vi "FPGA Main Default.vi"() -> ()   [LabVIEW 2019]
doc: "The myRIO v1.1 FPGA Shipping Personality. This personality contains support for:\n- 2 Analog Input Interrupt channel\n- 4 Digital Input Interrupt channel\n- 1 Timer\n- 1 Accelerometer\n- 1 Button\n- 4 LED\n- 10 Analog Input channels with 1 Sample\n- 6 Analog Output channels with 1 Sample\n- 40 Digital I/O channels with 1 Sample\n- 2 I2C channels\n- 4 Encoder channels\n- 6 PWM channels\n- 2 SPI channels"
uses:
  <vilib>/rvi/Emulation/niFpgaGetClockAttributes.vi
  <vilib>/rvi/Emulation/niFpgaSctlEmulationGetInTimedLoop.vi
  <vilib>/rvi/Emulation/niFpgaEmulationReportErrorSimple.vi
  <vilib>/rvi/Emulation/niFpgaProcessEmulError.vi
  <vilib>/rvi/eio/common/nirviEmuTemplateMethod_errors.vi
  <vilib>/rvi/Emulation/niFpgaCriticalErrorInLSC.vi
  <vilib>/eio/EIONode/EIONode.xnode
panel:
  in  "BreakinLoop":bool
  in  "OFFTime":u32
  in  "ONTime":u32
  in  "Trigger":u64
  in  "PulseNumberperLoop":i32
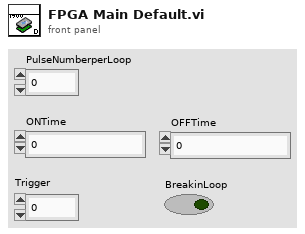
[diagram p1: front panel]
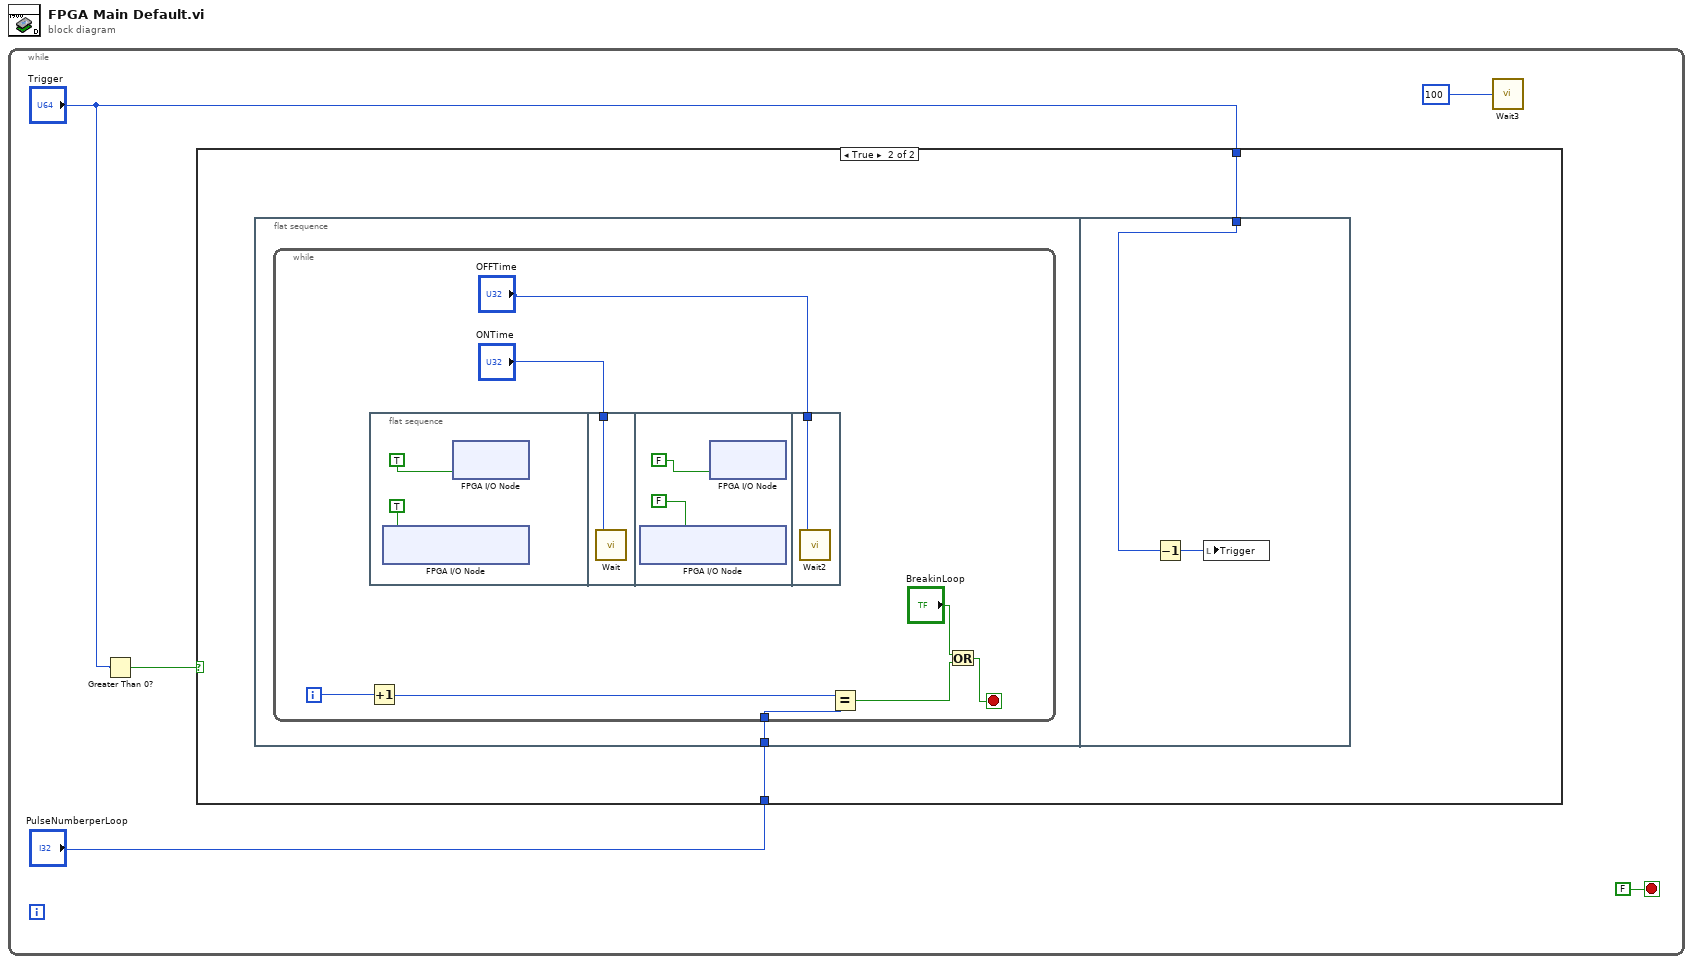
[diagram p0: block diagram]
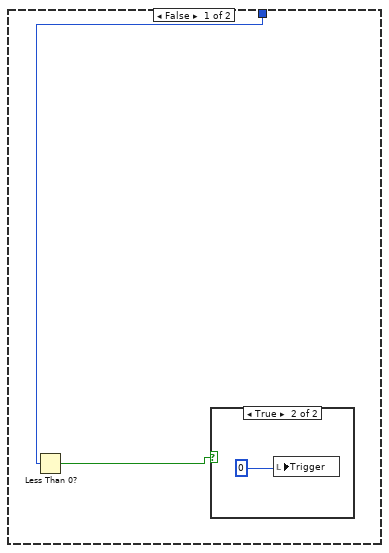
[diagram p2: hidden frame]
diagram:
  n1 = while {
    stop <- FALSE stop-if-true
    n2 = Greater Than 0?(x="Trigger") -> (x > 0?=w3:bool)
    n3 = case shown="True" w3 {
      tunnel: "PulseNumberperLoop" -> [_ w10]
      tunnel: "Trigger" -> [w7 w9]
      frame False {
        n4 = Less Than 0?(x=w7) -> (x < 0?=w6:bool)
        n5 = case shown="True" w6 {
          frame False {
          }
          frame True {
            n6 = local write "Trigger"(i16 0) -> ()
          }
        }
      }
      frame True {
        n7 = flat-sequence {
          tunnel: w10 -> [w11]
          tunnel: w9 -> [w26]
          frame #0 {
            n8 = while {
              tunnel: w11 -> [w12]
              i -> [w13]
              stop <- w17 stop-if-true
              n9 = Increment(x=w13) -> (x+1=w14:i32)
              n10 = flat-sequence {
                tunnel: "ONTime" -> [w22]
                tunnel: "OFFTime" -> [w25]
                frame #0 {
                  n11 = xnode "FPGA I/O Node"("ConnectorA/DIO8"=TRUE) -> ()  [unwired: 1 in, 1 out]
                  n12 = xnode "FPGA I/O Node"("LED0"=TRUE ("ConnectorA/DIO8")) -> ()  [unwired: 1 in, 1 out]
                }
                frame #1 {
                  n13 = call "Wait"("Count(uSec)"=w22) -> ()  [unwired: 1 out]
                }
                frame #2 {
                  n14 = xnode "FPGA I/O Node"("ConnectorA/DIO8"=FALSE) -> ()  [unwired: 1 in, 1 out]
                  n15 = xnode "FPGA I/O Node"("LED0"=FALSE ("ConnectorA/DIO8")) -> ()  [unwired: 1 in, 1 out]
                }
                frame #3 {
                  n16 = call "Wait2"("Count(uSec)"=w25) -> ()  [unwired: 1 out]
                }
              }
              n17 = Equal?(x=w14, y=w12) -> (x = y?=w19:bool)
              n18 = Or(x="BreakinLoop", y=w19) -> (x .or. y?=w17:bool)
            }
          }
          frame #1 {
            n19 = Decrement(x=w26) -> (x-1=w27:u64)
            n20 = local write "Trigger"(w27) -> ()
          }
        }
      }
    }
    n21 = call "Wait3"("Count(uSec)"=i16 100) -> ()  [unwired: 1 out]
  }
